vi "Save Data.vi"(0 "Experiment Indicator":string, 1 "Username":string, 5 "Pixel":dbl, 9 "Data Array":dbl[][](array[numeric]), 11 "Cell details cluster":T1={"Measure?"=TRUE, "Area (cm^2)"=0.0, "Cell Label"="", "Cell Description"="", "Cell Position"=0, "Time in rig (s)"=0.0, "Time to next scan (s)"=0.0, "Scan number"=0.0, "When did you stick it in?"=0.0, "Time between scans (s)"=0.0, "Time of the last scan (s)"=0.0, "Scan settings in queue"=0, "Sample Holder"=0.0} {"Scan settings in queue" items=["Regular", "Inverted"]; "Time of the last scan (s)" format="%<%H:%M:%S>t"; "When did you stick it in?" format="%<%H:%M:%S>t"; "Time to next scan (s)" format="%<%H:%M:%S>t"; "Time in rig (s)" format="%<%H:%M:%S>t"}, 12 "Show me Scan \nSettings JV set":T2={"Light Intensity (Suns)"=1.0, "Stabilization Time (s)"=5.0, "Maximum Voltage (V)"=0.0, "Minimum Voltage (V)"=-1.0, "Range Options"=0, "Scan Direction\nDU (T), UD (F)"=TRUE, "Step Size (V)"=0.01, "Source Delay (s)"=0.15} {"Range Options" items=["Auto Range", "Semi-Auto Range", "100 uA", "1 mA", "10 mA", "100 mA", "1A"]}, 13 "Time zero":timestamp) -> (4 "Master Log":string[][](table), 6 "File path for master log":path, 10 "File path for device log":path, 14 "File path for JV data":path, 15 "File path for JV image":path)   [LabVIEW 2013]
uses:
  <vilib>/Utility/file.llb/Write To Spreadsheet File (string).vi
  <vilib>/Utility/file.llb/Read From Spreadsheet File (string).vi
  <vilib>/Analysis/NI_AALPro.lvlib
panel:
  out "PCE":dbl
  out "FF":dbl
  out "Voc":dbl
  out "Jsc":dbl
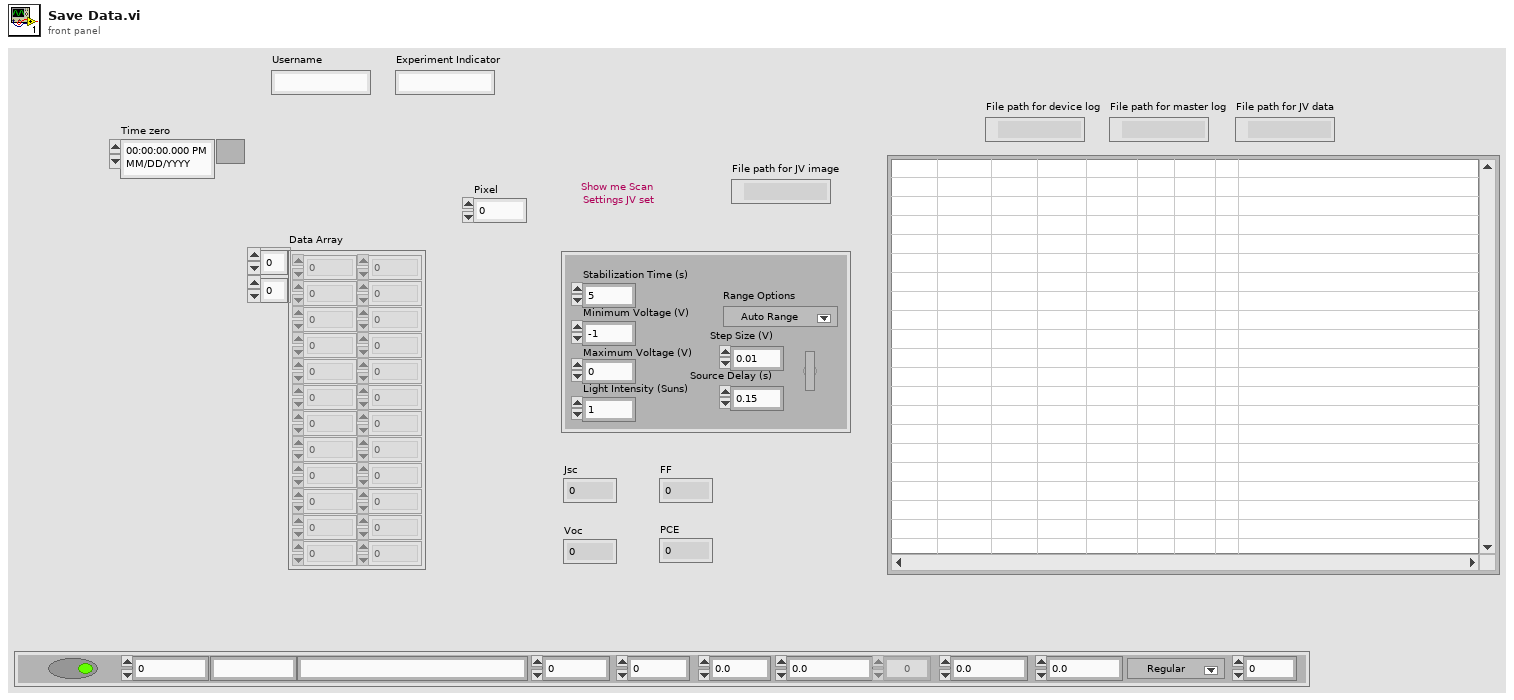
[diagram p1: front panel]
types:
  T1 = cluster{"Measure?":bool, "Area (cm^2)":dbl, "Cell Label":string, "Cell Description":string, "Cell Position":i32, "Time in rig (s)":dbl, "Time to next scan (s)":dbl, "Scan number":dbl, "When did you stick it in?":dbl, "Time between scans (s)":dbl, "Time of the last scan (s)":dbl, "Scan settings in queue":u16, "Sample Holder":dbl}
  T2 = cluster{"Light Intensity (Suns)":dbl, "Stabilization Time (s)":dbl, "Maximum Voltage (V)":dbl, "Minimum Voltage (V)":dbl, "Range Options":u16, "Scan Direction\nDU (T), UD (F)":bool, "Step Size (V)":dbl, "Source Delay (s)":dbl}
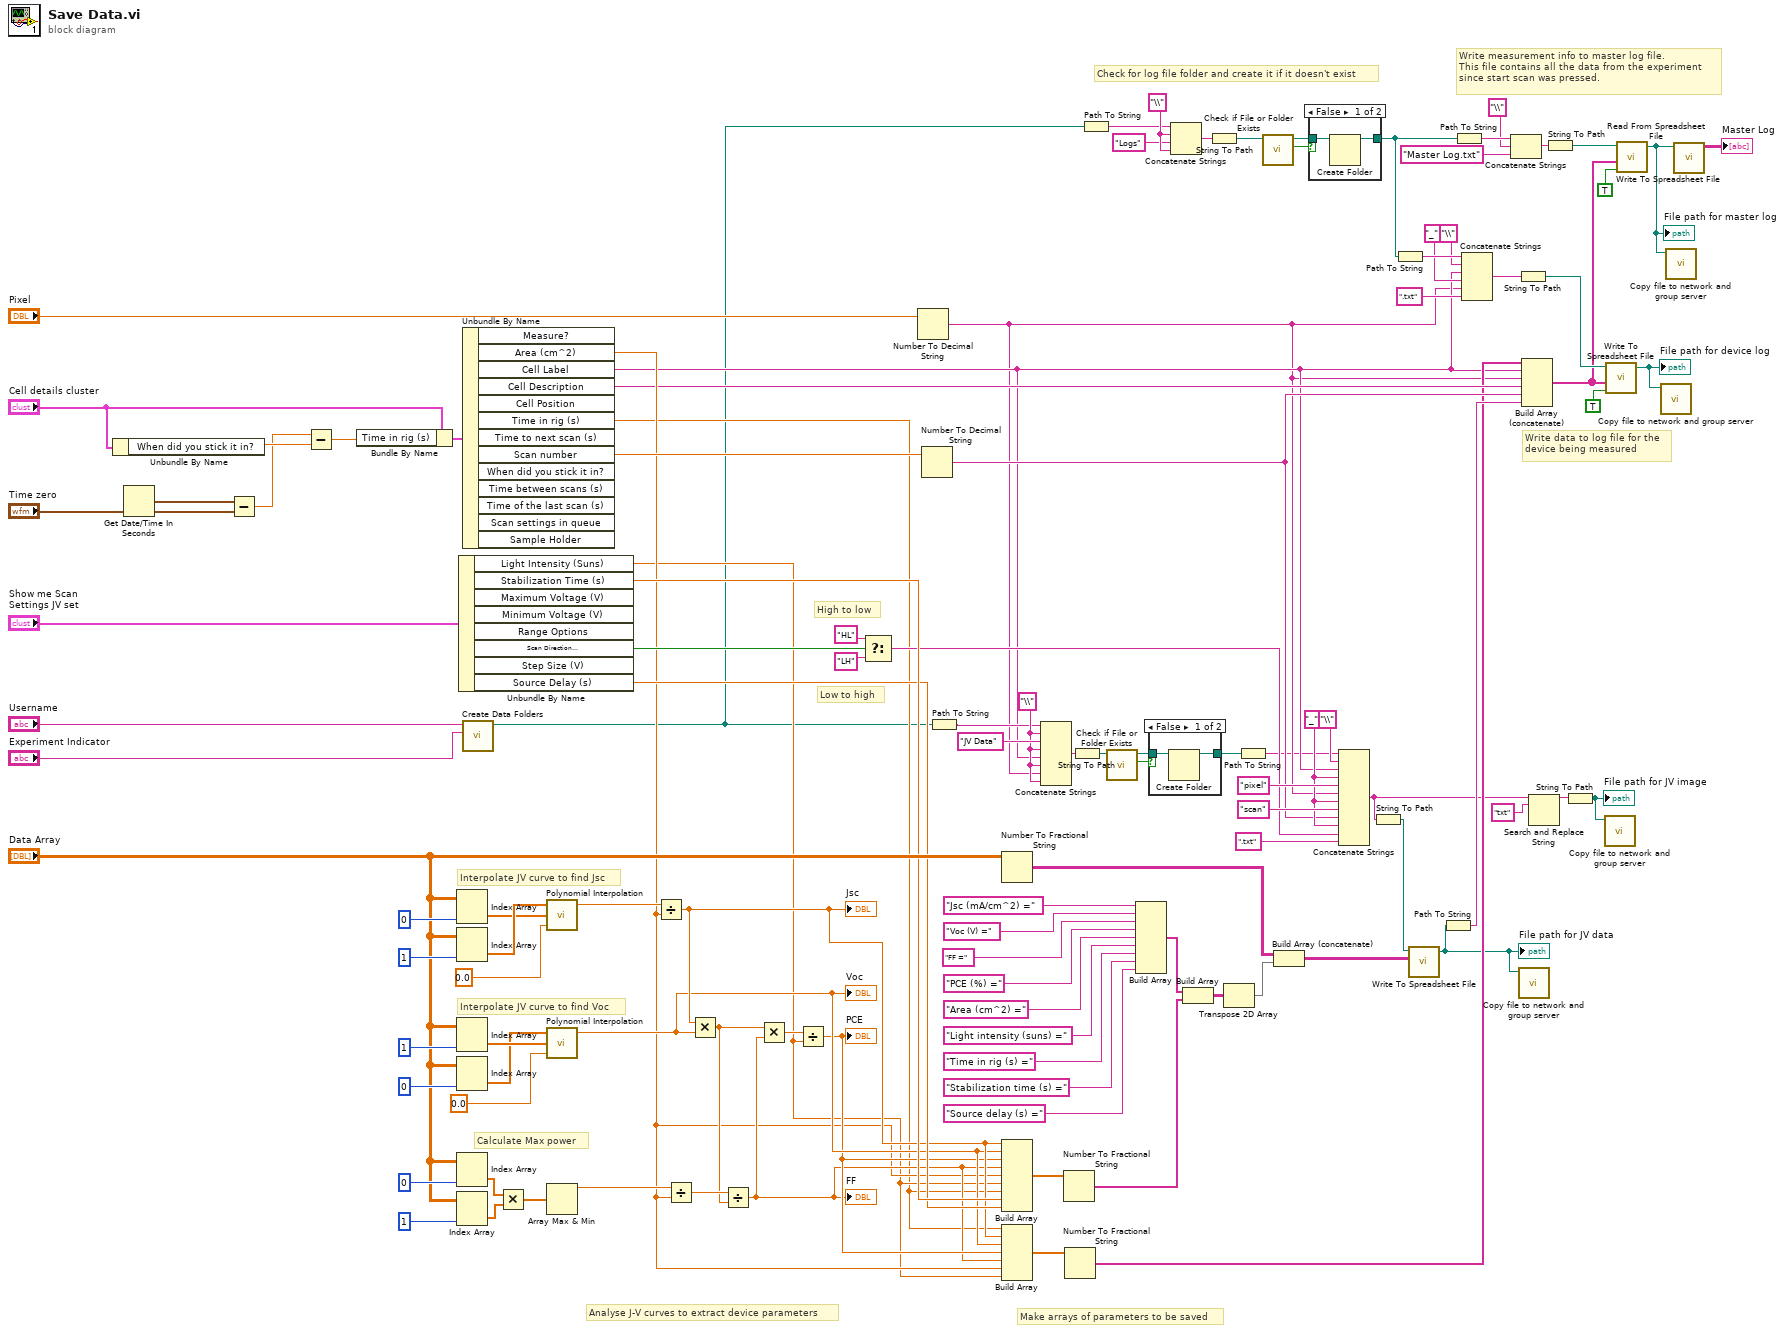
[diagram p0: block diagram]
diagram:
  w23 = "\\"
  w50 = "\\"
  w68 = "_"
  # "Make arrays of parameters to be saved"
  # "Calculate Max power"
  # "Interpolate JV curve to find Voc"
  # "Interpolate JV curve to find Jsc"
  # "Analyse J-V curves to extract device parameters"
  # "Write data to log file for the\ndevice being measured"
  # "Write measurement info to master log file.\nThis file contains all the data from the experiment\nsince start scan was pressed."
  # "Check for log file folder and create it if it doesn't exist"
  # "Low to high"
  # "High to low"
  n1 = Unbundle By Name("Cell details cluster") -> ("When did you stick it in?"=w5:dbl)
  n2 = Get Date/Time In Seconds() -> (seconds since 1Jan1904=w6:timestamp)
  n3 = Subtract(x=w6, y="Time zero") -> (x-y=w4:dbl)
  n4 = Subtract(x=w4, y=w5) -> (x-y=w2:dbl)
  n5 = Bundle By Name(cluster="Cell details cluster", "Time in rig (s)"=w2) -> (w7:T1)
  n6 = Index Array(array="Data Array", index (col)=0) -> (element=w101:dbl[])  [unwired: 1 in]
  n7 = Index Array(array="Data Array", index (col)=1) -> (element=w102:dbl[])  [unwired: 1 in]
  n8 = Index Array(array="Data Array", index (col)=1) -> (element=w100:dbl[])  [unwired: 1 in]
  n9 = Index Array(array="Data Array", index (col)=0) -> (element=w97:dbl[])  [unwired: 1 in]
  n10 = Index Array(array="Data Array", index (col)=0) -> (element=w108:dbl[])  [unwired: 1 in]
  n11 = Index Array(array="Data Array", index (col)=1) -> (element=w107:dbl[])  [unwired: 1 in]
  n12 = Unbundle By Name("Show me Scan \nSettings JV set") -> ("Light Intensity (Suns)"=w58:dbl, "Stabilization Time (s)"=w79:dbl, "Scan Direction\nDU (T), UD (F)"=w71:bool, "Source Delay (s)"=w78:dbl)  [unwired: 4 out]
  n13 = Unbundle By Name(w7) -> ("Area (cm^2)"=w59:dbl, "Cell Label"=w21:string, "Cell Description"=w56:string, "Time in rig (s)"=w57:dbl, "Scan number"=w74:dbl)  [unwired: 8 out]
  n14 = call "Create Data Folders.vi"("Experiment Indicator"="Experiment Indicator", "username"="Username") -> ("Data Output Folder"=w14:path)  [unwired: 9 in]
  n15 = Multiply(x=w108, y=w107) -> (x*y=w98:dbl[])
  n16 = call <vilib>:"Polynomial Interpolation.vi"("x value"=0.0, "X"=w101, "Y"=w102) -> ("interpolation value"=w105:dbl)  [unwired: 2 out]
  n17 = call <vilib>:"Polynomial Interpolation.vi"("x value"=0.0, "X"=w100, "Y"=w97) -> ("interpolation value"=w62:dbl)  [unwired: 2 out]
  "Voc" <- w62
  n18 = Array Max & Min(array=w98) -> (max value=w99:dbl)  [unwired: 3 out]
  n19 = Divide(x=w105, y=w59) -> (x/y=w63:dbl)
  "Jsc" <- w63
  n20 = Divide(x=w99, y=w59) -> (x/y=w96:dbl)
  n21 = Multiply(x=w63, y=w62) -> (x*y=w95:dbl)
  n22 = Divide(x=w96, y=w95) -> (x/y=w60:dbl)
  "FF" <- w60
  n23 = Multiply(x=w95, y=w60) -> (x*y=w106:dbl)
  n24 = Divide(x=w106, y=w58) -> (x/y=w61:dbl)
  "PCE" <- w61
  n25 = Select(t="HL", s=w71, f="LH") -> (s? t:f=w67:string)
  n26 = Number To Decimal String(number="Pixel") -> (decimal integer string=w20:string)  [unwired: 1 in]
  n27 = Number To Decimal String(number=w74) -> (decimal integer string=w55:string)  [unwired: 1 in]
  n28 = Path To String(path=w14) -> (string=w22:string)
  n29 = Number To Fractional String(number="Data Array") -> (F-format string=w86:string[][])  [unwired: 3 in]
  n30 = Build Array(w63, w62, w61, w60, w59, w58, w57, w79, w78) -> (w89:dbl[])
  n31 = Build Array(w57, w63, w62, w61, w60, w59, w58) -> (w53:dbl[])
  n32 = Concatenate Strings(w22, w23, "JV Data", w23, w21, w23, w20, w23) -> (w27:string)
  n33 = Number To Fractional String(number=w89) -> (F-format string=w87:string[])  [unwired: 3 in]
  n34 = Number To Fractional String(number=w53) -> (F-format string=w52:string[])  [unwired: 3 in]
  n35 = String To Path(string=w27) -> (path=w26:path)
  n36 = Path To String(path=w14) -> (string=w47:string)
  n37 = call <vilib>:"Check if File or Folder Exists.vi"("path"=w26) -> ("file or folder exists?"=w25:bool, "dup path"=w24:path)  [unwired: 8 in, 1 out]
  n38 = Build Array("Jsc (mA/cm^2) =", "Voc (V) =", "FF =", "PCE (%) =", "Area (cm^2) =", "Light intensity (suns) =", "Time in rig (s) =", "Stabilization time (s) =", "Source delay (s) =") -> (w88:string[])
  n39 = case shown="False" w25 {
    tunnel: w24 -> [w117 w118]
    tunnel: [w116 w118] -> w19
    frame False {
      n40 = Create Folder(path (use dialog)=w117) -> (created path=w116:path)  [unwired: 2 in, 2 out]
    }
    frame True {
    }
  }
  n41 = Concatenate Strings(w47, w50, "Logs", w50) -> (w48:string)
  n42 = Build Array(w88, w87) -> (w77:string[][])
  n43 = String To Path(string=w48) -> (path=w46:path)
  n44 = Transpose 2D Array(2D array=w77) -> (transposed array=w76:string[][])
  n45 = Path To String(path=w19) -> (string=w18:string)
  n46 = call <vilib>:"Check if File or Folder Exists.vi"("path"=w46) -> ("file or folder exists?"=w45:bool, "dup path"=w44:path)  [unwired: 8 in, 1 out]
  n47 = Build Array (concatenate)(w86, w76) -> (w85:string[][])
  n48 = case shown="False" w45 {
    tunnel: w44 -> [w120 w121]
    tunnel: [w119 w121] -> w37
    frame False {
      n49 = Create Folder(path (use dialog)=w120) -> (created path=w119:path)  [unwired: 2 in, 2 out]
    }
    frame True {
    }
  }
  n50 = Concatenate Strings(w18, "\\", w21, w68, "pixel", w20, w68, "scan", w55, w68, w67, ".txt") -> (w17:string)
  n51 = String To Path(string=w17) -> (path=w65:path)
  n52 = Path To String(path=w37) -> (string=w43:string)
  n53 = call-poly <vilib>:"Write To Spreadsheet File.vi"("2D data"=w85, "file path (dialog if empty)"=w65) -> ("new file path (Not A Path if cancelled)"=w10:path)  [unwired: 6 in]
  "File path for JV data" <- w10
  n54 = Path To String(path=w10) -> (string=w54:string)
  n55 = Path To String(path=w37) -> (string=w39:string)
  n56 = Concatenate Strings(w43, "\\", w21, "_", w20, ".txt") -> (w41:string)
  n57 = Concatenate Strings(w39, "\\", "Master Log.txt") -> (w35:string)
  n58 = String To Path(string=w41) -> (path=w40:path)
  n59 = call "Copy file to network and group server.vi"("File path in"=w10) -> ()  [unwired: 11 in]
  n60 = Build Array (concatenate)(w52, w21, w20, w56, w55, w54) -> (w33:string[])
  n61 = Search and Replace String(input string=w17, search string="txt") -> (result string=w16:string)  [unwired: 6 in, 3 out]
  n62 = String To Path(string=w35) -> (path=w34:path)
  n63 = String To Path(string=w16) -> (path=w11:path)
  "File path for JV image" <- w11
  n64 = call "Copy file to network and group server.vi"("File path in"=w11) -> ()  [unwired: 11 in]
  n65 = call-poly <vilib>:"Write To Spreadsheet File.vi"("append to file? (new file:F)"=TRUE, "1D data"=w33, "file path (dialog if empty)"=w40) -> ("new file path (Not A Path if cancelled)"=w9:path)  [unwired: 5 in]
  "File path for device log" <- w9
  n66 = call-poly <vilib>:"Write To Spreadsheet File.vi"("append to file? (new file:F)"=TRUE, "1D data"=w33, "file path (dialog if empty)"=w34) -> ("new file path (Not A Path if cancelled)"=w8:path)  [unwired: 5 in]
  "File path for master log" <- w8
  n67 = call "Copy file to network and group server.vi"("File path in"=w9) -> ()  [unwired: 11 in]
  n68 = call "Copy file to network and group server.vi"("File path in"=w8) -> ()  [unwired: 11 in]
  n69 = call-poly <vilib>:"Read From Spreadsheet File.vi"("file path (dialog if empty)"=w8) -> ("all rows"=→"Master Log":string[][])  [unwired: 6 in, 4 out]
